vi "Commands to ITX.vi"(1 "Commands":string) -> (0 "ITX Commands":string)   [LabVIEW 2019, in "ITX Commands.lvclass"]
uses:
  ITX Commands.lvclass
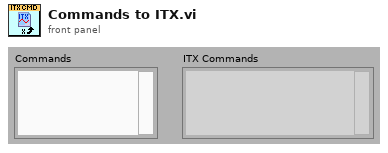
[diagram p1: front panel]
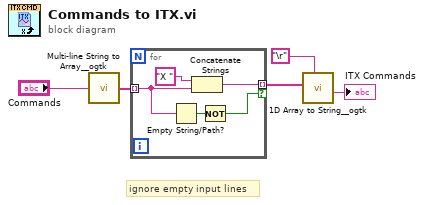
[diagram p0: block diagram]
diagram:
  # "ignore empty input lines"
  n1 = call "Multi-line String to Array__ogtk.vi"("string"="Commands") -> ("lines"=w3:string[])
  n2 = for {
    tunnel: w3 -> [w8] mode=indexing
    tunnel: [w9] -> w2 mode=indexing if=w6
    n3 = Empty String/Path?(string/path=w8) -> (empty?=w7:bool)
    n4 = Concatenate Strings("X " ("string"), w8) -> (w9:string)
    n5 = Not(x=w7) -> (.not. x?=w6:bool)
  }
  n6 = call "1D Array to String__ogtk.vi"("delimiter (Tab)"="\r", "Array of Strings"=w2) -> ("delimited string"=→"ITX Commands":string)  [unwired: 9 in]
